vi "R30_1-RT.vi"() -> ()   [LabVIEW 2016]
uses:
  GP307 cluster.ctl
  GV states.ctl
  Aperture states.ctl
  Faraday cup states.ctl
  Glassman Control.ctl
  <vilib>/Platform/TimedLoop/XDataNode/timing_clust.ctl
  <vilib>/Platform/TimedLoop/XDataNode/nitl_modes.ctl
  <vilib>/Platform/TimedLoop/XDataNode/wakeup.ctl
  <vilib>/FPGAPlugInAG/cRIO-9067/niLvFpga_Open_cRIO-9067.vi
  <vilib>/Utility/error.llb/Error Cluster From Error Code.vi
  <vilib>/rvi/errors/niLvFpgaAdjustHostInterfaceError.vi
  <vilib>/rvi/errors/niLvFpgaMergeErrorWithErrorCode.vi
  <vilib>/rvi/interface/nirviOpenFPGA/nirviOpenFPGA.xnode
  Slow-Switching-Control/FPGA Bitfiles/Controlsoftware2_FPGATarget9_R301-FPGA_M8vL--YnMbI.lvbitx
  R30_1-FPGA.vi
  <vilib>/Platform/TimedLoop/XDataNode/XDataNode.xnode
  <vilib>/rvi/interface/nirviReadWriteControl/nirviReadWriteControl.xnode
  Faraday Cup Readback.ctl
  Aperture Readback.ctl
  Gate Valve Readback.ctl
  <vilib>/Platform/TimedLoop/XDataNode/XDNodeRunTimeDep.lvlib
  NiFpgaLv.dll
panel:
  out "Error Reporter":errorcluster
  in  "Tab Control":enum32{"HV control", "Vacuum", "Actuators"}(tab)
  out "HV readback loop error":errorcluster
  out "ESA+ Monitor.I-monitor":fxp<+/-,26,5>
  out "ESA+ Monitor.V-monitor":fxp<+/-,26,7>
  out "ESA- Monitor.I-monitor":fxp<+/-,26,5>
  out "X- Steerer Monitor.V-monitor":fxp<+/-,26,7>
  out "Y+ Steerer Monitor.I-monitor":fxp<+/-,26,5>
  out "Y+ Steerer Monitor.V-monitor":fxp<+/-,26,7>
  out "Y- Steerer Monitor.I-monitor":fxp<+/-,26,5>
  out "Y- Steerer Monitor.V-monitor":fxp<+/-,26,7>
  out "Mag Steerer Monitor.I-monitor":fxp<+/-,26,5>
  out "Mag Steerer Monitor.V-monitor":fxp<+/-,26,7>
  out "X+ Steerer Monitor.V-monitor":fxp<+/-,26,7>
  out "ESA- Monitor.V-monitor":fxp<+/-,26,7>
  out "X- Steerer Monitor .I-monitor":fxp<+/-,26,5>
  out "Y+ Steerer V set":T1
  out "X+ Steerer Monitor.I-monitor":fxp<+/-,26,5>
  out "Quad B set":fxp<+/-,20,5>
  out "Quad A set":fxp<+/-,20,5>
  out "X- Steerer V set":T1
  out "Quad A I read":fxp<+/-,26,5>
  out "Quad B I read":fxp<+/-,26,5>
  out "X+ Steerer V set":T1
  out "Mag Steerer I-program":fxp<+/-,20,5>
  out "ESA Voltage set":fxp<+/-,20,5>
  out "ESA- HV Enable":bool
  out "ESA+ HV Enable":bool
  out "Y- Steerer V set":T1
  out "HV control loop error":errorcluster
  out "Vac cluster 3 Interlock":bool
  out "Vac cluster 2 Interlock":bool
  out "Vac cluster 1 Interlock":bool
  out "R30 Detector Ion gauge 1":u8[](array[numeric])
  out "R30 Detector Convectron  1":u8[](array[numeric])
  out "R30 ESA Ion gauge 1":u8[](array[numeric])
  out "Switch Image Convectron 1":u8[](array[numeric])
  out "Switch Image Ion Gauge 1":u8[](array[numeric])
  out "R30 ESA Convectron  1":u8[](array[numeric])
  out "Vac Cluster loop error":errorcluster
  out "Cryo 1st stage temp":u8[](array[numeric])
  out "Cryo On-time":u8[](array[numeric])
  out "Cryo status":u8[](array[numeric])
  out "Cryo 2nd stage temp":u8[](array[numeric])
  out "Time since repurge":u8[](array[numeric])
  out "Cryo loop error":errorcluster
  out "ESA Vac cluster":T2
  out "Switch Image Vac Cluster":T2
  out "Detector Vac Cluster":T2
  out "Interlock loop error":errorcluster
  out "Vac cluster 1 Interlock bypass":bool
  out "Vac cluster 2 Interlock bypass":bool
  out "Vac cluster 3 Interlock bypass":bool
  out "Switch Object Vac Interlock":bool
  out "Switch Object Interlock Bypass":bool
  out "Cryo Pump GV Status 2":T3
  out "Beamline GV 2 status 2":T3
  out "Turbo 2 GV status 2":T3
  out "Detector FC Status":T4
  out "Turbo 1 GV status 2":T3
  out "Switching Mag GV status 2":T3
  out "Switch Image FC Status":T4
  out "Switch Image Aperture Status":T5
  out "Beamline GV 1 status 2":T3
  out "Beamline GV 2 status":T6
  out "Turbo 2 GV status":T6
  out "Cryo Pump GV Status":T6
  out "Turbo 1 GV status":T6
  out "Switching Mag GV status":T6
  out "Detector FC Position":cluster{"IN sensor":bool, "OUT sensor":bool}
  out "Detector Aperture Status":T5
  out "Switch Image FC Position":cluster{"IN sensor":bool, "OUT sensor":bool}
  out "Switch Image Aperture Position":cluster{"IN sensor":bool, "OUT sensor":bool}
  out "Detector Aperture Position":cluster{"IN sensor":bool, "OUT sensor":bool}
  out "Actuator Sensor loop error":errorcluster
  out "Beamline GV 1 status":T6
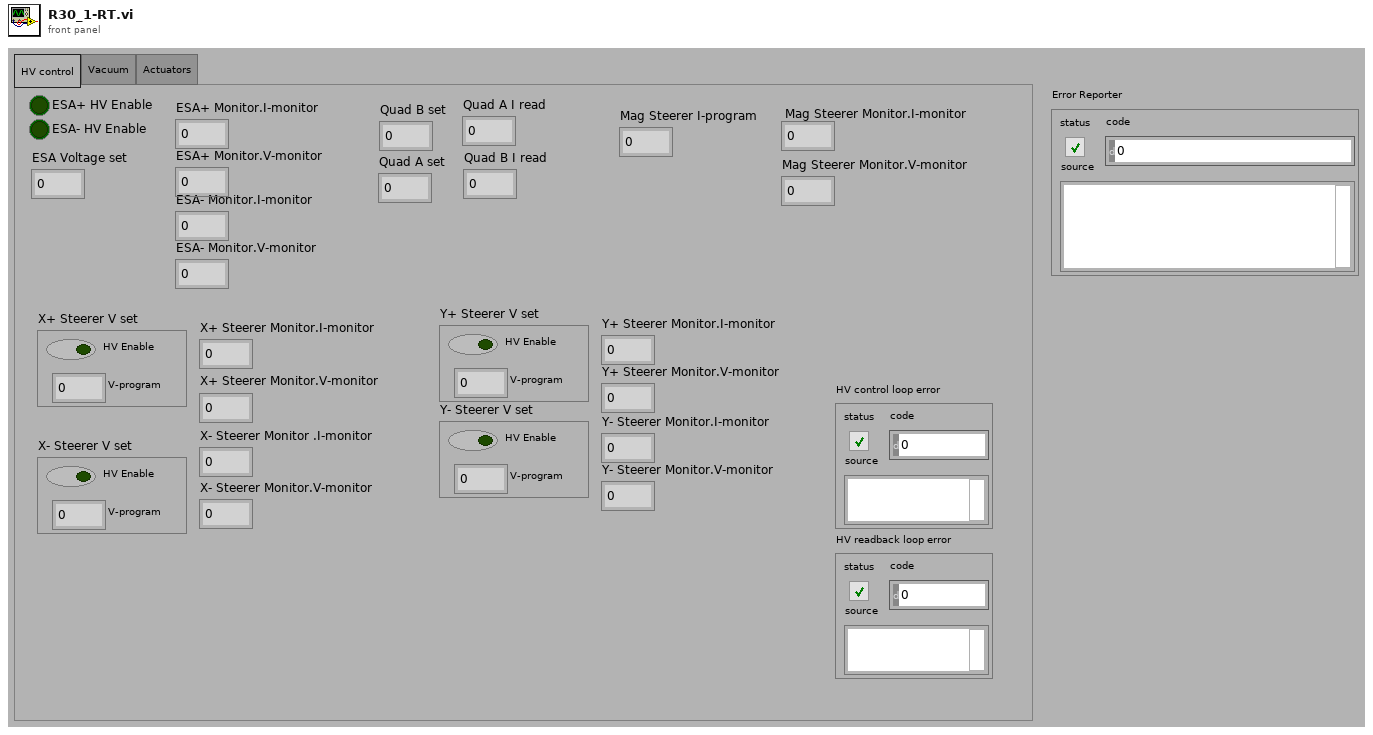
[diagram p1: front panel]
types:
  T1 = typedef "Glassman Control.ctl" = cluster{"V-program":fxp<+/-,20,5>, "HV Enable":bool}
  T2 = typedef "GP307 cluster.ctl" = cluster{"Ion gauge 1":string, "Convectron  Gauge 1 ":string, "Ion Gauge 2":string, "Convectrom Gauge 2":string}
  T3 = typedef "GV states.ctl" = enum16{"status unclear", "closed", "open"}
  T4 = typedef "Faraday cup states.ctl" = enum16{"FC status unclear", "FC in", "FC out"}
  T5 = typedef "Aperture states.ctl" = enum16{"Aperture status unclear", "Aperture in", "Aperture out"}
  T6 = cluster{"OPEN sensor":bool, "Closed sensor":bool}
  T7 = typedef "XDNodeRunTimeDep.lvlib/timing_clust.ctl" = cluster{"Expected End [f-1]":u64, "Actual End [f-1]":u64, "Finished Late? [f-1]":bool, "Expected End [i-1]":u64, "Actual End [i-1]":u64, "Finished Late? [i-1]":bool, "Expected Start [i]":u64, "Actual Start [i]":u64, "Expected Start [f]":u64, "Actual Start [f]":u64, "Source Name":string, "Structure Name":string, "Period":i64, "Deadline":i64, "Offset":i64, "Start":i64, "Priority":i32, "Timeout":i32, "Mode":T8, "Wakeup Reason":T9, "Error":errorcluster, "Source Type":string, "Secondary Source Type":string, "Global End Time":u64, "Global Start Time":u64, "Frame Duration":u64, "Iteration Duration":u64, "Assigned CPU":i32, "I/O Scan Engine Mode":u32}
  T8 = typedef "XDNodeRunTimeDep.lvlib/nitl_modes.ctl" = enum32{"No Change", "Process missed periods, maintain original phase", "Discard missed periods, maintain original phase", "Process missed periods, ignore original phase", "Discard missed periods, ignore original phase"}
  T9 = typedef "XDNodeRunTimeDep.lvlib/wakeup.ctl" = enum32{"Normal", "Aborted", "Asynchronous wakeup", "Timing source error", "Timed loop error", "Timeout"}
  T10 = typedef "Faraday Cup Readback.ctl" = cluster{"IN sensor":bool, "OUT sensor":bool}
  T11 = typedef "Aperture Readback.ctl" = cluster{"IN sensor":bool, "OUT sensor":bool}
  T12 = typedef "Gate Valve Readback.ctl" = cluster{"OPEN sensor":bool, "Closed sensor":bool}
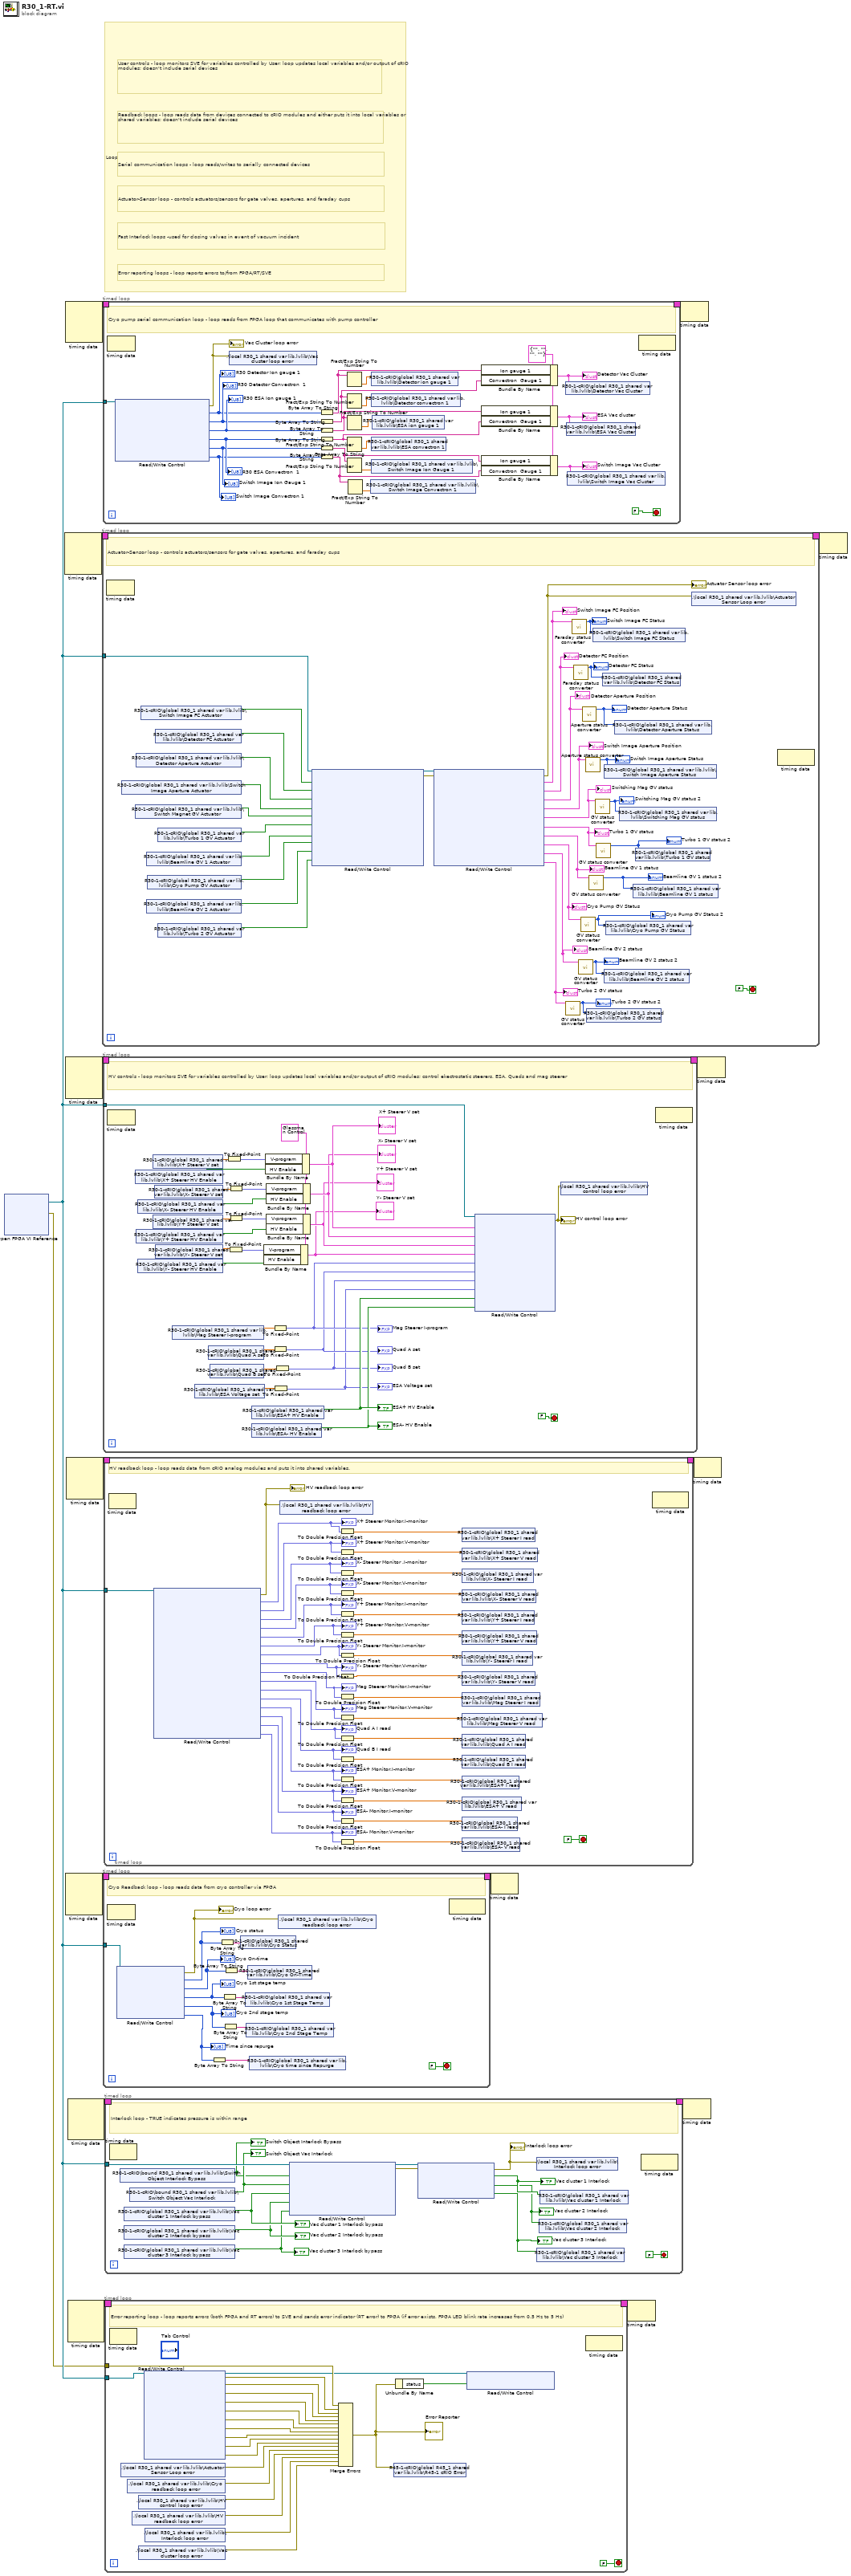
[diagram p0: block diagram]
diagram:
  # "Actuator-Sensor loop - controls actuators/sensors for gate valves, apertures, and faraday cups"
  # "Fast Interlock loops -used for closing valves in event of vacuum incident"
  # "Error reporting loops - loop reports errors to/from FPGA/RT/SVE"
  # "Serial communication loops - loop reads/writes to serially connected devices"
  # "Readback loops - loop reads data from devices connected to cRIO modules and either puts it into local variables or shared variables; doesn't include serial devices"
  # "User controls - loop monitors SVE for variables controlled by User; loop updates local variables and/or output of cRIO modules; doesn't include serial devices"
  # "Loop legend - loops are color coded by responsibility"
  n1 = xnode "Open FPGA VI Reference"() -> ("FPGA VI Reference Out"=w2:refnum<k20>, "error out"=w1:errorcluster)  [unwired: 2 in]
  n2 = node-c288() -> (w14:T7)  [unwired: 4 in]
  n3 = node-c288() -> (w16:T7)  [unwired: 4 in]
  n4 = node-c288() -> (w12:T7)  [unwired: 4 in]
  n5 = node-c288() -> (w8:T7)  [unwired: 4 in]
  n6 = node-c288() -> (w10:T7)  [unwired: 4 in]
  n7 = node-c288() -> (w6:T7)  [unwired: 4 in]
  n8 = node-c288() -> (w4:T7)  [unwired: 4 in]
  n9 = timed-loop {
    tunnel: w2 -> [w17]
    timing: w14 -> [_]
    timing-out: [_] -> w13
    stop <- FALSE stop-if-true
    # "Actuator-Sensor loop - controls actuators/sensors for gate valves, apertures, and faraday cups"
    n10 = node-c288() -> ()  [unwired: 1 in, 1 out]
    n11 = shared-variable "R30-1-cRIO\\global R30_1 shared var lib.lvlib\\Switch Image Aperture Actuator"() -> (w44:bool)  [unwired: 1 in, 1 out]
    n12 = shared-variable "R30-1-cRIO\\global R30_1 shared var lib.lvlib\\Switch Magnet GV Actuator"() -> (w28:bool)  [unwired: 1 in, 1 out]
    n13 = shared-variable "R30-1-cRIO\\global R30_1 shared var lib.lvlib\\Detector Aperture Actuator"() -> (w45:bool)  [unwired: 1 in, 1 out]
    n14 = shared-variable "R30-1-cRIO\\global R30_1 shared var lib.lvlib\\Switch Image FC Actuator"() -> (w47:bool)  [unwired: 1 in, 1 out]
    n15 = shared-variable "R30-1-cRIO\\global R30_1 shared var lib.lvlib\\Beamline GV 1 Actuator"() -> (w24:bool)  [unwired: 1 in, 1 out]
    n16 = shared-variable "R30-1-cRIO\\global R30_1 shared var lib.lvlib\\Beamline GV 2 Actuator"() -> (w26:bool)  [unwired: 1 in, 1 out]
    n17 = shared-variable "R30-1-cRIO\\global R30_1 shared var lib.lvlib\\Cryo Pump GV Actuator"() -> (w25:bool)  [unwired: 1 in, 1 out]
    n18 = shared-variable "R30-1-cRIO\\global R30_1 shared var lib.lvlib\\Detector FC Actuator"() -> (w46:bool)  [unwired: 1 in, 1 out]
    n19 = shared-variable "R30-1-cRIO\\global R30_1 shared var lib.lvlib\\Turbo 1 GV Actuator"() -> (w23:bool)  [unwired: 1 in, 1 out]
    n20 = shared-variable "R30-1-cRIO\\global R30_1 shared var lib.lvlib\\Turbo 2 GV Actuator"() -> (w27:bool)  [unwired: 1 in, 1 out]
    n21 = xnode "Read/Write Control"("FPGA VI Reference In"=w17, "Switch magnet FC Actuator"=w47, "Detector FC Actuator"=w46, "Detector Aperture Actuator"=w45, "Switch magnet Aperture Actuator"=w44, "Switch Magnet GV Actuator"=w28, "Turbo 1 GV Actuator"=w23, "Beamline GV 1 Actuator"=w24, "Cryo Pump GV Actuator"=w25, "Beamline GV 2 Actuator"=w26, "Turbo 2 GV Actuator"=w27) -> ("FPGA VI Reference Out"=w50:refnum<k20>, "error out"=w49:errorcluster)  [unwired: 1 in]
    n22 = xnode "Read/Write Control"("FPGA VI Reference In"=w50, "error in"=w49) -> ("error out"=w48:errorcluster, "Switch Magnet FC Position"=w29:T10, "Detector FC Position"=w31:T10, "Detector Aperture Position"=w30:T11, "Switch Magnet Aperture Position"=w33:T11, "Switching Mag GV Status"=w36:T12, "Turbo 1 GV Status"=w37:T12, "Beamline GV 1 Status"=w18:T12, "Cryo Pump GV Status"=w35:T12, "Beamline GV 2 Status"=w20:T12, "Turbo 2 GV Status"=w34:T12)  [unwired: 1 out]
    "Actuator Sensor loop error" <- w48
    "Beamline GV 1 status" <- w18
    "Switch Image FC Position" <- w29
    "Switch Image Aperture Position" <- w33
    "Cryo Pump GV Status" <- w35
    "Beamline GV 2 status" <- w20
    "Turbo 2 GV status" <- w34
    "Turbo 1 GV status" <- w37
    "Switching Mag GV status" <- w36
    "Detector Aperture Position" <- w30
    "Detector FC Position" <- w31
    n23 = call "GV status converter.vi"("Gate Valve"=w34) -> ("GV Status"=w21:T3)  [unwired: 10 in]
    "Turbo 2 GV status 2" <- w21
    n24 = call "Faraday status converter.vi"("FC Position"=w29) -> ("FC Status"=w42:T4)  [unwired: 10 in]
    "Switch Image FC Status" <- w42
    n25 = call "Faraday status converter.vi"("FC Position"=w31) -> ("FC Status"=w22:T4)  [unwired: 10 in]
    "Detector FC Status" <- w22
    n26 = call "GV status converter.vi"("Gate Valve"=w20) -> ("GV Status"=w40:T3)  [unwired: 10 in]
    "Beamline GV 2 status 2" <- w40
    n27 = call "GV status converter.vi"("Gate Valve"=w35) -> ("GV Status"=w41:T3)  [unwired: 10 in]
    "Cryo Pump GV Status 2" <- w41
    n28 = call "Aperture status converter.vi"("Aperture Position"=w30) -> ("Aperture Status"=w32:T5)  [unwired: 10 in]
    "Detector Aperture Status" <- w32
    n29 = call "Aperture status converter.vi"("Aperture Position"=w33) -> ("Aperture Status"=w43:T5)  [unwired: 10 in]
    "Switch Image Aperture Status" <- w43
    n30 = shared-variable "R30-1-cRIO\\global R30_1 shared var lib.lvlib\\Turbo 2 GV status"(w21) -> ()  [unwired: 1 in, 1 out]
    n31 = call "GV status converter.vi"("Gate Valve"=w18) -> ("GV Status"=w19:T3)  [unwired: 10 in]
    "Beamline GV 1 status 2" <- w19
    n32 = shared-variable "R30-1-cRIO\\global R30_1 shared var lib.lvlib\\Switch Image FC Status"(w42) -> ()  [unwired: 1 in, 1 out]
    n33 = call "GV status converter.vi"("Gate Valve"=w36) -> ("GV Status"=w38:T3)  [unwired: 10 in]
    "Switching Mag GV status 2" <- w38
    n34 = call "GV status converter.vi"("Gate Valve"=w37) -> ("GV Status"=w39:T3)  [unwired: 10 in]
    "Turbo 1 GV status 2" <- w39
    n35 = shared-variable "R30-1-cRIO\\global R30_1 shared var lib.lvlib\\Detector FC Status"(w22) -> ()  [unwired: 1 in, 1 out]
    n36 = shared-variable "R30-1-cRIO\\global R30_1 shared var lib.lvlib\\Beamline GV 2 status"(w40) -> ()  [unwired: 1 in, 1 out]
    n37 = shared-variable "R30-1-cRIO\\global R30_1 shared var lib.lvlib\\Switch Image Aperture Status"(w43) -> ()  [unwired: 1 in, 1 out]
    n38 = shared-variable "R30-1-cRIO\\global R30_1 shared var lib.lvlib\\Cryo Pump GV Status"(w41) -> ()  [unwired: 1 in, 1 out]
    n39 = shared-variable "R30-1-cRIO\\global R30_1 shared var lib.lvlib\\Detector Aperture Status"(w32) -> ()  [unwired: 1 in, 1 out]
    n40 = shared-variable "R30-1-cRIO\\global R30_1 shared var lib.lvlib\\Switching Mag GV status"(w38) -> ()  [unwired: 1 in, 1 out]
    n41 = shared-variable "R30-1-cRIO\\global R30_1 shared var lib.lvlib\\Beamline GV 1 status"(w19) -> ()  [unwired: 1 in, 1 out]
    n42 = shared-variable "R30-1-cRIO\\global R30_1 shared var lib.lvlib\\Turbo 1 GV status"(w39) -> ()  [unwired: 1 in, 1 out]
    n43 = shared-variable ".\\local R30_1 shared var lib.lvlib\\Actuator Sensor Loop error"(w48) -> ()  [unwired: 1 in, 1 out]
    n44 = node-c288() -> ()  [unwired: 1 in, 1 out]
  }
  n45 = timed-loop {
    tunnel: w2 -> [w78]
    timing: w16 -> [_]
    timing-out: [_] -> w15
    stop <- FALSE stop-if-true
    w68 = T2 {"Ion gauge 1"="", "Convectron  Gauge 1 "="", "Ion Gauge 2"="", "Convectrom Gauge 2"=""} ("Ion gauge cluster control")
    # "Cryo pump serial communication loop - loop reads from FPGA loop that communicates with pump controller"
    n46 = node-c288() -> ()  [unwired: 1 in, 1 out]
    n47 = xnode "Read/Write Control"("FPGA VI Reference In"=w78) -> ("error out"=w54:errorcluster, "R30 Detector Ion gauge 1"=w73:u8[], "R30 Detector Convectron  1"=w74:u8[], "R30 ESA Ion gauge 1"=w75:u8[], "R30 ESA Convectron  1"=w76:u8[], "Switch Image Ion Gauge 1"=w67:u8[], "Switch Image Convectron 1"=w66:u8[])  [unwired: 1 in, 1 out]
    "R30 Detector Ion gauge 1" <- w73
    "R30 Detector Convectron  1" <- w74
    "R30 ESA Ion gauge 1" <- w75
    "Switch Image Convectron 1" <- w66
    "Switch Image Ion Gauge 1" <- w67
    "R30 ESA Convectron  1" <- w76
    "Vac Cluster loop error" <- w54
    n48 = shared-variable ".\\local R30_1 shared var lib.lvlib\\Vac cluster loop error"(w54) -> ()  [unwired: 1 in, 1 out]
    n49 = Byte Array To String(unsigned byte array=w73) -> (string=w65:string)
    n50 = Byte Array To String(unsigned byte array=w74) -> (string=w64:string)
    n51 = Byte Array To String(unsigned byte array=w75) -> (string=w63:string)
    n52 = Byte Array To String(unsigned byte array=w76) -> (string=w62:string)
    n53 = Byte Array To String(unsigned byte array=w67) -> (string=w59:string)
    n54 = Byte Array To String(unsigned byte array=w66) -> (string=w58:string)
    n55 = Fract/Exp String To Number(string=w65) -> (number=w70:dbl)  [unwired: 3 in, 1 out]
    n56 = Fract/Exp String To Number(string=w64) -> (number=w69:dbl)  [unwired: 3 in, 1 out]
    n57 = Fract/Exp String To Number(string=w63) -> (number=w72:dbl)  [unwired: 3 in, 1 out]
    n58 = Fract/Exp String To Number(string=w62) -> (number=w71:dbl)  [unwired: 3 in, 1 out]
    n59 = Fract/Exp String To Number(string=w59) -> (number=w61:dbl)  [unwired: 3 in, 1 out]
    n60 = Fract/Exp String To Number(string=w58) -> (number=w60:dbl)  [unwired: 3 in, 1 out]
    n61 = shared-variable "R30-1-cRIO\\global R30_1 shared var lib.lvlib\\Switch Image Convectron 1"(w60) -> ()  [unwired: 1 in, 1 out]
    n62 = shared-variable "R30-1-cRIO\\global R30_1 shared var lib.lvlib\\Detector ion gauge 1"(w70) -> ()  [unwired: 1 in, 1 out]
    n63 = shared-variable "R30-1-cRIO\\global R30_1 shared var lib.lvlib\\Detector convectron 1"(w69) -> ()  [unwired: 1 in, 1 out]
    n64 = shared-variable "R30-1-cRIO\\global R30_1 shared var lib.lvlib\\ESA convectron 1"(w71) -> ()  [unwired: 1 in, 1 out]
    n65 = shared-variable "R30-1-cRIO\\global R30_1 shared var lib.lvlib\\Switch Image Ion Gauge 1"(w61) -> ()  [unwired: 1 in, 1 out]
    n66 = shared-variable "R30-1-cRIO\\global R30_1 shared var lib.lvlib\\ESA ion gauge 1"(w72) -> ()  [unwired: 1 in, 1 out]
    n67 = Bundle By Name(cluster=w68, "Ion gauge 1"=w65, "Convectron  Gauge 1"=w64) -> (w55:T2)
    "Detector Vac Cluster" <- w55
    n68 = Bundle By Name(cluster=w68, "Ion gauge 1"=w63, "Convectron  Gauge 1"=w62) -> (w56:T2)
    "ESA Vac cluster" <- w56
    n69 = Bundle By Name(cluster=w68, "Ion gauge 1"=w59, "Convectron  Gauge 1"=w58) -> (w57:T2)
    "Switch Image Vac Cluster" <- w57
    n70 = shared-variable "R30-1-cRIO\\global R30_1 shared var lib.lvlib\\Detector Vac Cluster"(w55) -> ()  [unwired: 1 in, 1 out]
    n71 = shared-variable "R30-1-cRIO\\global R30_1 shared var lib.lvlib\\ESA Vac Cluster"(w56) -> ()  [unwired: 1 in, 1 out]
    n72 = shared-variable "R30-1-cRIO\\global R30_1 shared var lib.lvlib\\Switch Image Vac Cluster"(w57) -> ()  [unwired: 1 in, 1 out]
    n73 = node-c288() -> ()  [unwired: 1 in, 1 out]
  }
  n74 = timed-loop {
    tunnel: w2 -> [w99]
    timing: w12 -> [_]
    timing-out: [_] -> w11
    stop <- FALSE stop-if-true
    w86 = T1 {"V-program"=0.0, "HV Enable"=FALSE} ("Glassman Control")
    # "HV controls - loop monitors SVE for variables controlled by User; loop updates local variables and/or output of cRIO modules; control ekectrostatic steerers, ESA, Quads and mag steerer"
    n75 = node-c288() -> ()  [unwired: 1 in, 1 out]
    n76 = shared-variable "R30-1-cRIO\\global R30_1 shared var lib.lvlib\\X+ Steerer HV Enable"() -> (w88:bool)  [unwired: 1 in, 1 out]
    n77 = shared-variable "R30-1-cRIO\\global R30_1 shared var lib.lvlib\\Y+ Steerer HV Enable"() -> (w90:bool)  [unwired: 1 in, 1 out]
    n78 = shared-variable "R30-1-cRIO\\global R30_1 shared var lib.lvlib\\X- Steerer HV Enable"() -> (w89:bool)  [unwired: 1 in, 1 out]
    n79 = shared-variable "R30-1-cRIO\\global R30_1 shared var lib.lvlib\\Y- Steerer HV Enable"() -> (w95:bool)  [unwired: 1 in, 1 out]
    n80 = shared-variable "R30-1-cRIO\\global R30_1 shared var lib.lvlib\\X+ Steerer V set"() -> (w91:dbl)  [unwired: 1 in, 1 out]
    n81 = shared-variable "R30-1-cRIO\\global R30_1 shared var lib.lvlib\\Y+ Steerer V set"() -> (w94:dbl)  [unwired: 1 in, 1 out]
    n82 = shared-variable "R30-1-cRIO\\global R30_1 shared var lib.lvlib\\X- Steerer V set"() -> (w92:dbl)  [unwired: 1 in, 1 out]
    n83 = shared-variable "R30-1-cRIO\\global R30_1 shared var lib.lvlib\\Y- Steerer V set"() -> (w96:dbl)  [unwired: 1 in, 1 out]
    n84 = shared-variable "R30-1-cRIO\\global R30_1 shared var lib.lvlib\\Mag Steerer I-program"() -> (w109:dbl)  [unwired: 1 in, 1 out]
    n85 = shared-variable "R30-1-cRIO\\global R30_1 shared var lib.lvlib\\ESA Voltage set"() -> (w101:dbl)  [unwired: 1 in, 1 out]
    n86 = shared-variable "R30-1-cRIO\\global R30_1 shared var lib.lvlib\\Quad A set"() -> (w105:dbl)  [unwired: 1 in, 1 out]
    n87 = shared-variable "R30-1-cRIO\\global R30_1 shared var lib.lvlib\\Quad B set"() -> (w103:dbl)  [unwired: 1 in, 1 out]
    n88 = To Fixed-Point(number=w91) -> (fixed-point=w87:fxp<+/-,20,7>)  [unwired: 1 in]
    n89 = To Fixed-Point(number=w96) -> (fixed-point=w98:fxp<+/-,20,7>)  [unwired: 1 in]
    n90 = To Fixed-Point(number=w92) -> (fixed-point=w97:fxp<+/-,20,7>)  [unwired: 1 in]
    n91 = To Fixed-Point(number=w94) -> (fixed-point=w93:fxp<+/-,20,7>)  [unwired: 1 in]
    n92 = shared-variable "R30-1-cRIO\\global R30_1 shared var lib.lvlib\\ESA+ HV Enable"() -> (w108:bool)  [unwired: 1 in, 1 out]
    "ESA+ HV Enable" <- w108
    n93 = shared-variable "R30-1-cRIO\\global R30_1 shared var lib.lvlib\\ESA- HV Enable"() -> (w107:bool)  [unwired: 1 in, 1 out]
    "ESA- HV Enable" <- w107
    n94 = Bundle By Name(cluster=w86, "V-program"=w98, "HV Enable"=w95) -> (w82:T1)
    "Y- Steerer V set" <- w82
    n95 = Bundle By Name(cluster=w86, "V-program"=w87, "HV Enable"=w88) -> (w85:T1)
    "X+ Steerer V set" <- w85
    n96 = Bundle By Name(cluster=w86, "V-program"=w97, "HV Enable"=w89) -> (w84:T1)
    "X- Steerer V set" <- w84
    n97 = Bundle By Name(cluster=w86, "V-program"=w93, "HV Enable"=w90) -> (w83:T1)
    "Y+ Steerer V set" <- w83
    n98 = To Fixed-Point(number=w109) -> (fixed-point=w106:fxp<+/-,20,5>)  [unwired: 1 in]
    "Mag Steerer I-program" <- w106
    n99 = To Fixed-Point(number=w105) -> (fixed-point=w104:fxp<+/-,20,5>)  [unwired: 1 in]
    "Quad A set" <- w104
    n100 = To Fixed-Point(number=w101) -> (fixed-point=w100:fxp<+/-,20,5>)  [unwired: 1 in]
    "ESA Voltage set" <- w100
    n101 = To Fixed-Point(number=w103) -> (fixed-point=w102:fxp<+/-,20,5>)  [unwired: 1 in]
    "Quad B set" <- w102
    n102 = xnode "Read/Write Control"("FPGA VI Reference In"=w99, "X+ Steerer V set"=w85, "X- Steerer V set"=w84, "Y+ Steerer V set"=w83, "Y- Steerer V set"=w82, "Mag Steerer I-program"=w106, "Quad A set"=w104, "Quad B set"=w102, "ESA Voltage set"=w100, "ESA+ HV Enable"=w108, "ESA- HV Enable"=w107) -> ("error out"=w81:errorcluster)  [unwired: 1 in, 1 out]
    "HV control loop error" <- w81
    n103 = shared-variable ".\\local R30_1 shared var lib.lvlib\\HV control loop error"(w81) -> ()  [unwired: 1 in, 1 out]
    n104 = node-c288() -> ()  [unwired: 1 in, 1 out]
  }
  n105 = timed-loop {
    timing: w8 -> [_]
    timing-out: [_] -> w7
    tunnel: w2 -> [w124]
    stop <- FALSE stop-if-true
    # "Cryo Readback loop - loop reads data from cryo controller via FPGA"
    n106 = node-c288() -> ()  [unwired: 1 in, 1 out]
    n107 = xnode "Read/Write Control"("FPGA VI Reference In"=w124) -> ("error out"=w117:errorcluster, "Cryo Status"=w121:u8[], "Cryo On-time"=w122:u8[], "1st stage temp"=w123:u8[], "2nd stage temp"=w120:u8[], "Time since repurge"=w119:u8[])  [unwired: 1 in, 1 out]
    "Cryo status" <- w121
    "Cryo On-time" <- w122
    "Cryo 1st stage temp" <- w123
    "Cryo loop error" <- w117
    "Cryo 2nd stage temp" <- w120
    "Time since repurge" <- w119
    n108 = Byte Array To String(unsigned byte array=w119) -> (string=w116:string)
    n109 = Byte Array To String(unsigned byte array=w121) -> (string=w118:string)
    n110 = Byte Array To String(unsigned byte array=w123) -> (string=w114:string)
    n111 = Byte Array To String(unsigned byte array=w120) -> (string=w115:string)
    n112 = Byte Array To String(unsigned byte array=w122) -> (string=w113:string)
    n113 = shared-variable "R30-1-cRIO\\global R30_1 shared var lib.lvlib\\Cryo Status"(w118) -> ()  [unwired: 1 in, 1 out]
    n114 = shared-variable "R30-1-cRIO\\global R30_1 shared var lib.lvlib\\Cryo 1st Stage Temp"(w114) -> ()  [unwired: 1 in, 1 out]
    n115 = shared-variable "R30-1-cRIO\\global R30_1 shared var lib.lvlib\\Cryo 2nd Stage Temp"(w115) -> ()  [unwired: 1 in, 1 out]
    n116 = shared-variable "R30-1-cRIO\\global R30_1 shared var lib.lvlib\\Cryo On-Time"(w113) -> ()  [unwired: 1 in, 1 out]
    n117 = shared-variable "R30-1-cRIO\\global R30_1 shared var lib.lvlib\\Cryo time since Repurge"(w116) -> ()  [unwired: 1 in, 1 out]
    n118 = shared-variable ".\\local R30_1 shared var lib.lvlib\\Cryo readback loop error"(w117) -> ()  [unwired: 1 in, 1 out]
    n119 = node-c288() -> ()  [unwired: 1 in, 1 out]
  }
  n120 = timed-loop {
    timing: w10 -> [_]
    timing-out: [_] -> w9
    tunnel: w2 -> [w161]
    stop <- FALSE stop-if-true
    # "HV readback loop - loop reads data from cRIO analog modules and puts it into shared variables."
    n121 = node-c288() -> ()  [unwired: 1 in, 1 out]
    n122 = xnode "Read/Write Control"("FPGA VI Reference In"=w161) -> ("error out"=w160:errorcluster, "X+ Steerer Monitor.I-monitor"=w159:fxp<+/-,26,5>, "X+ Steerer Monitor.V-monitor"=w158:fxp<+/-,26,7>, "X- Steerer Monitor .I-monitor"=w157:fxp<+/-,26,5>, "X- Steerer Monitor .V-monitor"=w156:fxp<+/-,26,7>, "Y+ Steerer Monitor.I-monitor"=w155:fxp<+/-,26,5>, "Y+ Steerer Monitor.V-monitor"=w154:fxp<+/-,26,7>, "Y- Steerer Monitor.I-monitor"=w153:fxp<+/-,26,5>, "Y- Steerer Monitor.V-monitor"=w152:fxp<+/-,26,7>, "Mag Steerer Monitor.I-monitor"=w151:fxp<+/-,26,5>, "Mag Steerer Monitor.V-monitor"=w150:fxp<+/-,26,7>, "Quad A I read"=w149:fxp<+/-,26,5>, "Quad B I read"=w148:fxp<+/-,26,5>, "ESA+ Monitor.I-monitor"=w147:fxp<+/-,26,5>, "ESA+ Monitor.V-monitor"=w146:fxp<+/-,26,7>, "ESA- Monitor.I-monitor"=w145:fxp<+/-,26,5>, "ESA- Monitor.V-monitor"=w144:fxp<+/-,26,7>)  [unwired: 1 in, 1 out]
    "HV readback loop error" <- w160
    "X+ Steerer Monitor.I-monitor" <- w159
    "X+ Steerer Monitor.V-monitor" <- w158
    "X- Steerer Monitor .I-monitor" <- w157
    "X- Steerer Monitor.V-monitor" <- w156
    "Y+ Steerer Monitor.I-monitor" <- w155
    "Y+ Steerer Monitor.V-monitor" <- w154
    "Y- Steerer Monitor.I-monitor" <- w153
    "Y- Steerer Monitor.V-monitor" <- w152
    "Mag Steerer Monitor.I-monitor" <- w151
    "Mag Steerer Monitor.V-monitor" <- w150
    "Quad A I read" <- w149
    "Quad B I read" <- w148
    "ESA+ Monitor.I-monitor" <- w147
    "ESA+ Monitor.V-monitor" <- w146
    "ESA- Monitor.I-monitor" <- w145
    "ESA- Monitor.V-monitor" <- w144
    n123 = shared-variable ".\\local R30_1 shared var lib.lvlib\\HV readback loop error"(w160) -> ()  [unwired: 1 in, 1 out]
    n124 = To Double Precision Float(number=w159) -> (double precision float=w128:dbl)
    n125 = To Double Precision Float(number=w158) -> (double precision float=w129:dbl)
    n126 = To Double Precision Float(number=w157) -> (double precision float=w130:dbl)
    n127 = To Double Precision Float(number=w156) -> (double precision float=w131:dbl)
    n128 = To Double Precision Float(number=w155) -> (double precision float=w132:dbl)
    n129 = To Double Precision Float(number=w154) -> (double precision float=w133:dbl)
    n130 = To Double Precision Float(number=w153) -> (double precision float=w134:dbl)
    n131 = To Double Precision Float(number=w152) -> (double precision float=w135:dbl)
    n132 = To Double Precision Float(number=w151) -> (double precision float=w143:dbl)
    n133 = To Double Precision Float(number=w150) -> (double precision float=w142:dbl)
    n134 = To Double Precision Float(number=w149) -> (double precision float=w141:dbl)
    n135 = To Double Precision Float(number=w148) -> (double precision float=w140:dbl)
    n136 = To Double Precision Float(number=w147) -> (double precision float=w139:dbl)
    n137 = To Double Precision Float(number=w146) -> (double precision float=w138:dbl)
    n138 = To Double Precision Float(number=w145) -> (double precision float=w137:dbl)
    n139 = To Double Precision Float(number=w144) -> (double precision float=w136:dbl)
    n140 = shared-variable "R30-1-cRIO\\global R30_1 shared var lib.lvlib\\X+ Steerer I read"(w128) -> ()  [unwired: 1 in, 1 out]
    n141 = shared-variable "R30-1-cRIO\\global R30_1 shared var lib.lvlib\\X+ Steerer V read"(w129) -> ()  [unwired: 1 in, 1 out]
    n142 = shared-variable "R30-1-cRIO\\global R30_1 shared var lib.lvlib\\X- Steerer I read"(w130) -> ()  [unwired: 1 in, 1 out]
    n143 = shared-variable "R30-1-cRIO\\global R30_1 shared var lib.lvlib\\X- Steerer V read"(w131) -> ()  [unwired: 1 in, 1 out]
    n144 = shared-variable "R30-1-cRIO\\global R30_1 shared var lib.lvlib\\Y+ Steerer I read"(w132) -> ()  [unwired: 1 in, 1 out]
    n145 = shared-variable "R30-1-cRIO\\global R30_1 shared var lib.lvlib\\Y+ Steerer V read"(w133) -> ()  [unwired: 1 in, 1 out]
    n146 = shared-variable "R30-1-cRIO\\global R30_1 shared var lib.lvlib\\Y- Steerer I read"(w134) -> ()  [unwired: 1 in, 1 out]
    n147 = shared-variable "R30-1-cRIO\\global R30_1 shared var lib.lvlib\\Y- Steerer V read"(w135) -> ()  [unwired: 1 in, 1 out]
    n148 = shared-variable "R30-1-cRIO\\global R30_1 shared var lib.lvlib\\Mag Steerer I read"(w143) -> ()  [unwired: 1 in, 1 out]
    n149 = shared-variable "R30-1-cRIO\\global R30_1 shared var lib.lvlib\\Mag Steerer V read"(w142) -> ()  [unwired: 1 in, 1 out]
    n150 = shared-variable "R30-1-cRIO\\global R30_1 shared var lib.lvlib\\Quad A I read"(w141) -> ()  [unwired: 1 in, 1 out]
    n151 = shared-variable "R30-1-cRIO\\global R30_1 shared var lib.lvlib\\Quad B I read"(w140) -> ()  [unwired: 1 in, 1 out]
    n152 = shared-variable "R30-1-cRIO\\global R30_1 shared var lib.lvlib\\ESA+ I read"(w139) -> ()  [unwired: 1 in, 1 out]
    n153 = shared-variable "R30-1-cRIO\\global R30_1 shared var lib.lvlib\\ESA+ V read"(w138) -> ()  [unwired: 1 in, 1 out]
    n154 = shared-variable "R30-1-cRIO\\global R30_1 shared var lib.lvlib\\ESA- I read"(w137) -> ()  [unwired: 1 in, 1 out]
    n155 = shared-variable "R30-1-cRIO\\global R30_1 shared var lib.lvlib\\ESA- V read"(w136) -> ()  [unwired: 1 in, 1 out]
    n156 = node-c288() -> ()  [unwired: 1 in, 1 out]
  }
  n157 = timed-loop {
    timing: w6 -> [_]
    timing-out: [_] -> w5
    tunnel: w2 -> [w177]
    stop <- FALSE stop-if-true
    # "Interlock loop - TRUE indicates pressure is within range"
    n158 = node-c288() -> ()  [unwired: 1 in, 1 out]
    n159 = shared-variable "R30-1-cRIO\\bound R30_1 shared var lib.lvlib\\Switch Object Interlock Bypass"() -> (w165:bool)  [unwired: 1 in, 1 out]
    "Switch Object Interlock Bypass" <- w165
    n160 = shared-variable "R30-1-cRIO\\global R30_1 shared var lib.lvlib\\Vac cluster 1 Interlock bypass"() -> (w168:bool)  [unwired: 1 in, 1 out]
    "Vac cluster 1 Interlock bypass" <- w168
    n161 = shared-variable "R30-1-cRIO\\global R30_1 shared var lib.lvlib\\Vac cluster 2 Interlock bypass"() -> (w167:bool)  [unwired: 1 in, 1 out]
    "Vac cluster 2 Interlock bypass" <- w167
    n162 = shared-variable "R30-1-cRIO\\global R30_1 shared var lib.lvlib\\Vac cluster 3 Interlock bypass"() -> (w166:bool)  [unwired: 1 in, 1 out]
    "Vac cluster 3 Interlock bypass" <- w166
    n163 = shared-variable "R30-1-cRIO\\bound R30_1 shared var lib.lvlib\\Switch Object Vac Interlock"() -> (w169:bool)  [unwired: 1 in, 1 out]
    "Switch Object Vac Interlock" <- w169
    n164 = xnode "Read/Write Control"("FPGA VI Reference In"=w177, "Switch Obj Vac interlock bypass"=w165, "Switch Object Vac Interlock"=w169, "Vac cluster 1 interlock bypass"=w168, "Vac cluster 2 interlock bypass"=w167, "Vac cluster 3 interlock bypass"=w166) -> ("FPGA VI Reference Out"=w171:refnum<k20>, "error out"=w170:errorcluster)  [unwired: 1 in]
    n165 = xnode "Read/Write Control"("FPGA VI Reference In"=w171, "error in"=w170) -> ("error out"=w172:errorcluster, "Vac cluster 1 Interlock"=w174:bool, "Vac cluster 2 Interlock"=w173:bool, "Vac cluster 3 Interlock"=w175:bool)  [unwired: 1 out]
    "Interlock loop error" <- w172
    "Vac cluster 1 Interlock" <- w174
    "Vac cluster 2 Interlock" <- w173
    "Vac cluster 3 Interlock" <- w175
    n166 = shared-variable "R30-1-cRIO\\global R30_1 shared var lib.lvlib\\Vac cluster 3 Interlock"(w175) -> ()  [unwired: 1 in, 1 out]
    n167 = shared-variable ".\\local R30_1 shared var lib.lvlib\\Interlock loop error"(w172) -> ()  [unwired: 1 in, 1 out]
    n168 = shared-variable "R30-1-cRIO\\global R30_1 shared var lib.lvlib\\Vac cluster 2 Interlock"(w173) -> ()  [unwired: 1 in, 1 out]
    n169 = shared-variable "R30-1-cRIO\\global R30_1 shared var lib.lvlib\\Vac cluster 1 Interlock"(w174) -> ()  [unwired: 1 in, 1 out]
    n170 = node-c288() -> ()  [unwired: 1 in, 1 out]
  }
  n171 = timed-loop {
    timing: w4 -> [_]
    timing-out: [_] -> w3
    tunnel: w2 -> [w201]
    tunnel: w1 -> [w200]
    stop <- FALSE stop-if-true
    # "Error reporting loop - loop reports errors (both FPGA and RT errors) to SVE and sends error indicator (RT error) to FPGA (if error exists, FPGA LED blink rate increases from 0.5 Hz to 5 Hz)"
    n172 = node-c288() -> ()  [unwired: 1 in, 1 out]
    n173 = shared-variable ".\\local R30_1 shared var lib.lvlib\\Actuator Sensor Loop error"() -> (w185:errorcluster)  [unwired: 1 in, 1 out]
    n174 = shared-variable ".\\local R30_1 shared var lib.lvlib\\Cryo readback loop error"() -> (w184:errorcluster)  [unwired: 1 in, 1 out]
    n175 = shared-variable ".\\local R30_1 shared var lib.lvlib\\HV readback loop error"() -> (w182:errorcluster)  [unwired: 1 in, 1 out]
    n176 = shared-variable ".\\local R30_1 shared var lib.lvlib\\HV control loop error"() -> (w183:errorcluster)  [unwired: 1 in, 1 out]
    n177 = shared-variable ".\\local R30_1 shared var lib.lvlib\\Vac cluster loop error"() -> (w180:errorcluster)  [unwired: 1 in, 1 out]
    n178 = xnode "Read/Write Control"("FPGA VI Reference In"=w201) -> ("FPGA VI Reference Out"=w190:refnum<k20>, "error out"=w199:errorcluster, "Vacuum Gauge 1 error"=w198:errorcluster, "Vacuum Gauge 2 error"=w197:errorcluster, "Vacuum Gauge 1 error"=w196:errorcluster, "Cryo Readback error"=w195:errorcluster, "HV control loop error"=w194:errorcluster, "Actuator loop error"=w193:errorcluster, "GV Status Loop error"=w192:errorcluster, "GV Interlock loop error"=w187:errorcluster, "HV readback loop error"=w186:errorcluster)  [unwired: 1 in]
    n179 = shared-variable ".\\local R30_1 shared var lib.lvlib\\Interlock loop error"() -> (w181:errorcluster)  [unwired: 1 in, 1 out]
    n180 = Merge Errors(w200, w199, w198, w197, w196, w195, w194, w193, w192, w187, w186, w185, w184, w183, w182, w181, w180) -> (w191:errorcluster)
    "Error Reporter" <- w191
    n181 = shared-variable "R45-1-cRIO\\global R45_1 shared var lib.lvlib\\R45-1 cRIO Error"(w191) -> ()  [unwired: 1 in, 1 out]
    n182 = Unbundle By Name(w191) -> ("status"=w189:bool)
    n183 = xnode "Read/Write Control"("FPGA VI Reference In"=w190, "RT error"=w189) -> ()  [unwired: 1 in, 2 out]
    n184 = node-c288() -> ()  [unwired: 1 in, 1 out]
  }
  n185 = node-c288(w7) -> ()  [unwired: 1 out]
  n186 = node-c288(w3) -> ()  [unwired: 1 out]
  n187 = node-c288(w15) -> ()  [unwired: 1 out]
  n188 = node-c288(w5) -> ()  [unwired: 1 out]
  n189 = node-c288(w9) -> ()  [unwired: 1 out]
  n190 = node-c288(w11) -> ()  [unwired: 1 out]
  n191 = node-c288(w13) -> ()  [unwired: 1 out]
